vi "Write Open Thermocouple Detection.vi"(8 "error in":errorcluster, 10 "open thermocouple detection":bool, 11 "NI 9213 in":refnum<class "NI 9213.lvclass">) -> (0 "error out":errorcluster, 3 "NI 9213 out":refnum<class "NI 9213.lvclass">)   [LabVIEW 2019, in "Scan Engine Scripting.lvlib" / "NI 9213.lvclass"]
uses:
  NI 9213.lvclass
  NI 9213.lvclass/NI 9213.ctl
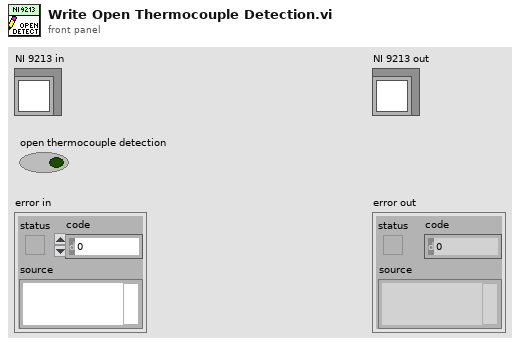
[diagram p1: front panel]
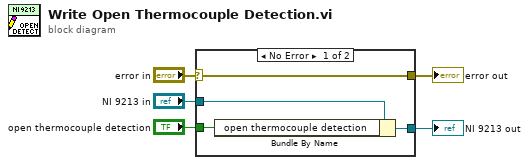
[diagram p0: block diagram]
diagram:
  n1 = case shown="No Error" "error in" {
    selector: "error in" -> [w9 w10]
    tunnel: [w9 w10] -> w4
    tunnel: [w7 w11] -> w1
    tunnel: "NI 9213 in" -> [w8 w11]
    tunnel: "open thermocouple detection" -> [w6 _]
    frame No Error {
      n2 = Bundle By Name(cluster=w8, "open thermocouple detection"=w6) -> (w7:refnum<class "NI 9213.lvclass">)
    }
    frame Error {
    }
  }
  "error out" <- w4
  "NI 9213 out" <- w1
